vi "Generate Waveform.vi"(8 "error in":errorcluster, 11 "Generator in":refnum<class "GeneradorAmplificado.lvclass">) -> (0 "error out":errorcluster, 3 "Generator out":refnum<class "GeneradorAmplificado.lvclass">)   [LabVIEW 2020, in "FGen.lvlib" / "GeneradorAmplificado.lvclass"]
uses:
  Generador/Generador.lvclass/Generador.ctl
  Generador/Set amplitude.vi
  Generador/Set frequency.vi
  Generador/Set offset.vi
  Generador/Set phase.vi
  Generador/Set sampling info.vi
  Generador/Set square wave duty cycle (%).vi
  GeneradorAmplificado.lvclass
  Generador/Generador.lvclass
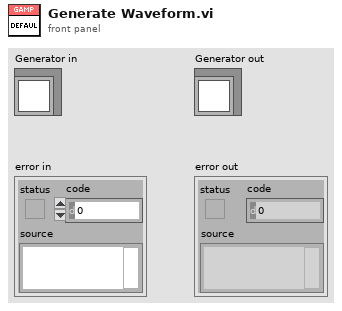
[diagram p1: front panel]
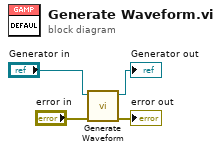
[diagram p0: block diagram]
diagram:
  n1 = call-parent "Generate Waveform.vi"("error in"="error in", "Generator in"="Generator in") -> ("error out"=→"error out":errorcluster, "Generator out"=→"Generator out":refnum<class "GeneradorAmplificado.lvclass">)  [unwired: 8 in]
